vi "TemperatureControl.vi"() -> ()   [LabVIEW 2019]
panel:
  in  "TemperatureTab":enum32{"Temperature Panel", "Setup"}(tab)
  in  "ChangeTemp":bool
  in  "Set Point (K)":dbl=4.2 format="%.2f"
  out "Temperature History(K)":dbl(graph)
  in  "Temperature Parameters":T1={"LTC-GPIB Address"=7, "Temp Tolerance"=1.0, "LTC-20?"=FALSE, "Mode?"=FALSE, "Magneto Correction?"=FALSE, "Advance?"=FALSE} {"Temp Tolerance" format="%.2f"; "LTC-GPIB Address" min=2 max=31 step=1}
  in  "LTC20 Cal Table?":bool
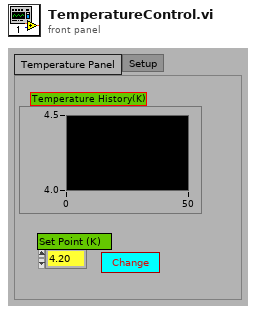
[diagram p1: front panel]
types:
  T1 = cluster{"LTC-GPIB Address":i16, "Temp Tolerance":dbl, "LTC-20?":bool, "Mode?":bool, "Magneto Correction?":bool, "Advance?":bool}
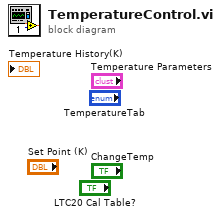
[diagram p0: block diagram]
diagram:
